vi "Xctrl interface-Set X axis multiplier.vi"(8 "error in (no error)":errorcluster) -> (0 "error out":errorcluster)   [LabVIEW 2020]
uses:
  XGrapher.xctl
  Global variables/gl_Functional Imaging-Global variables.vi
  SubVIs/Experiment header interface/Typedefs/Header file interface module functions enum.ctl
  Typedefs/Get-Set-Clear Control.ctl
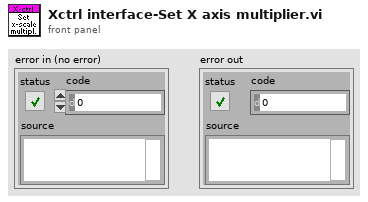
[diagram p1: front panel]
types:
  T1 = typedef "Get-Set-Clear Control.ctl" = enum16{"Get", "Set", "Clear"}
  T2 = typedef "Header file interface module functions enum.ctl" = enum16{"Load experiment header file", "Save experiment header file", "Clear stored values", "Read stored values", "Update specific value in memory", "Update values in memory"}
  T3 = typedef "Header parameters cluster-ALL.ctl" = cluster{"LOGIN":T4, "GLOBAL PARAMETERS":T5, "IMAGING MODES":T7, "TIME SERIES":T8, "MOTOR Z-STACK ":T11, "AOL Z-STACK":T12, "FUNCTIONAL IMAGING":T13, "VOLUME IMAGING":T13, "MOVEMENT CORRECTION":T17, "CALIBRATION":T19, "STATISTICS":T20, "BIOLOGY INFORMATION":T21, "Calibration Data":T22}
  T4 = typedef "Header params -Login.ctl" = cluster{"User":string, "Profile":string, "Software Version":string, "Experiment Date Time":timestamp}
  T5 = typedef "Header params-Global Parameters.ctl" = cluster{"MicroscopeID":string, "Microscope Type":string, "Objective":string, "Field of View (um)":dbl, "Fill time (us)":dbl, "Experiment Type":T6, "Stimuli Trigger":bool, "Speed Logging":bool}
  T6 = typedef "Experiment Type.ctl" = enum16{"In vivo", "In vitro", "Testing", "Calibration", "Other"}
  T7 = typedef "Header params-Imaging Modes.ctl" = cluster{"Time Series":bool, "Motor Zstack":bool, "AOL Zstack":bool, "Functional Imaging":bool, "Volume Imaging":bool}
  T8 = typedef "Header params-Time Series.ctl" = cluster{"Basic Image meta data":T9, "AOL z":dbl}
  T9 = typedef "Header params-Basic image meta data.ctl" = cluster{"Wavelength (nm)":dbl, "# averaged frames":dbl, "laser power (%)":dbl, "Pockels":dbl, "pixel dwell time (us)":dbl, "pmt 1":dbl, "pmt 2":dbl, "back apperture":dbl, "zoom":dbl, "field of view":dbl, "Frame Size":T10, "AOL x centre":dbl, "AOL y centre":dbl, "Stage x position":dbl, "Stage y position":dbl, "Stage z position":dbl}
  T10 = typedef "Frame Size.ctl" = u16
  T11 = typedef "Header params-Motor Z-stack.ctl" = cluster{"Hdr Basic Image meta data":T9, "Z Start":dbl, "Z Stop":dbl, "No of Planes":i32, "Laser Power (%) at Z Start":dbl, "Laser Power (%) at Z Stop":dbl}
  T12 = typedef "Header params-AOL Z-stack.ctl" = cluster{"Hdr Basic Image meta data":T9, "Z Start":dbl, "Z Stop":dbl, "No of Planes":i32, "Laser Power (%) at Z Start":dbl, "Laser Power (%) at Z Stop":dbl}
  T13 = typedef "Header params-Functional Imaging.ctl" = cluster{"Functional Mode":T14, "Variable Length":bool, "Variable Resolution":bool, "Pockels Modulation":bool, "Stimuli Trigger":bool, "Cool down enabled":bool, "AOL Mode":T15, "Plane Mode":T16, "Miniscan Dwell time per pixel (us)":dbl, "poi dwell time":dbl, "Number of trials":dbl, "Number of cycles":dbl, "Number of pois":dbl, "Number of miniscans":dbl, "Number of pixels in miniscan":dbl, "Rectangle ROI length":dbl, "Rectangle ROI height":dbl, "Frame rate (fps)":dbl, "Acquisition Length":dbl, "video length (sec)":dbl, "Stimuli delay (sec)":dbl, "Cool down time (sec)":dbl, "Basic Image meta data":T9, "Z Start (um)":dbl, "Z Stop (um)":dbl}
  T14 = typedef "Functional Mode.ctl" = enum16{"Point", "Line", "Patch", "Plane", "Volume"}
  T15 = typedef "AOL modes.ctl" = enum16{"Raster", "Structural", "Pointing", "Mini Scan", "Alignment"}
  T16 = typedef "Plane Mode.ctl" = u16
  T17 = typedef "Header params-Movement correction.ctl" = cluster{"Movement Correction":bool, "Axial Reference":bool, "Reference Source":T18, "Full Frame Size":dbl, "Reference Field of View":dbl, "Reference Zoom":dbl, "Reference dwell time (us)":dbl, "Reference X Pixels":dbl, "Reference Y Pixels":dbl, "Number of Z lines":dbl, "Size of Z pixels":dbl, "Axial Pixels":dbl, "Ignore Z lines":dbl, "Reference Scan Cycles":dbl, "Reference Threshold XY":dbl, "Reference Threshold Z":dbl, "Reference Average XY":dbl, "Reference Average Z":dbl, "Proportional Scale":dbl, "Integral Scale":dbl, "Proportional Scale Z":dbl, "Integral Scale Z":dbl, "Diff Threshold":dbl, "Diff Threshold Z":dbl, "Sliding Average":bool, "Reference count reset enabled":bool, "Scan Interval (ms)":dbl, "Ref Plot Refresh Rate (ms)":dbl}
  T18 = typedef "Reference source.ctl" = enum16{"Green channel", "Red channel"}
  T19 = typedef "Header params-Calibration Setup.ctl" = cluster{"Pockels Calibration File":path, "Calibration_ini file":path, "Setup_ini file":path}
  T20 = typedef "Header params-statistics.ctl" = cluster{"Z-stack duration (sec)":dbl, "Number of acquired data-points":dbl, "Acquisition time (ms)":dbl, "Number of acquired frames":dbl, "Intertrial times":dbl[]}
  T21 = typedef "Biology Information.ctl" = cluster{"Animal Code or Name":string, "Animal DoB":string, "Animal Age":string, "Animal Sex":string, "Animal Weight":string, "Date of Injection":string, "Date of Implant":string, "Site of Injection":string, "Animal Ear Notch":string, "AAV constructs":string, "Genetic background":string, "Optical reporter":string, "Region of brain imaged":string, "Other \ncomments":string}
  T22 = typedef "Header params-calibration data.ctl" = cluster{"Objective Name":string, "Calibration Wavelength":dbl, "Sum X":dbl, "Sum Y":dbl, "Diff X":dbl, "Diff Y":dbl, "Distortion Correction":dbl, " Z norm to um Scaling":dbl, " X norm to um Scaling":dbl}
  T23 = typedef "Functional Imging UI Refs.ctl" = cluster{"Menu ref":refnum<k9>, "Image control":refnum<vi>, "VI ref":refnum<vi>, "XGrapher":refnum<vi>, "Smoothing":refnum<vi>, "POI Averaging":refnum<vi>, "Normalize":refnum<vi>, "POI data points in each trial":refnum<vi>, "Channel":refnum<vi>, "Experiment data folder path":refnum<vi>, "[ROI vis]":refnum<vi>, "[Groups] visbl":T24, "Group Name":refnum<vi>, "POI index":refnum<vi>, "Trial No.":refnum<vi>, "Intensity Zoom":refnum<vi>, "Trial Cursor Enabled":refnum<vi>, "Number of Trials (ind 1)":refnum<vi>, "Number of Trials (ind 2)":refnum<vi>, "MiniScans Available":refnum<vi>, "POI Available":refnum<vi>, "Defer graph updates":refnum<vi>, "Waveform selector":refnum<vi>, "#of selected POI":refnum<vi>, "#of selected MiniScans":refnum<vi>, "#of selected groups":refnum<vi>, "Max Z-Projection":refnum<vi>, "Z-Plane Selector":refnum<vi>, "Index of miniscan point to visualise":refnum<vi>, "ROI vis. mode":refnum<vi>, "Total # of points":refnum<vi>, "Index of group clicked on":refnum<vi>, "Pane 1":refnum<vi>, "Pane 2":refnum<vi>, "Pane 3":refnum<vi>, "Pane 4":refnum<vi>, "Pane 5":refnum<vi>, "Pane 6":refnum<vi>, "Deselect all ROI":refnum<vi>, "Deselect all groups":refnum<vi>}
  T24 = typedef "Groups array referecne.ctl" = refnum<vi>
  T25 = typedef "XGrapher.xctl/Xctrl-Waveform graph ref.ctl" = refnum<vi>
  T26 = typedef "XGrapher.xctl/Xctrl-Timeline graph ref.ctl" = refnum<vi>
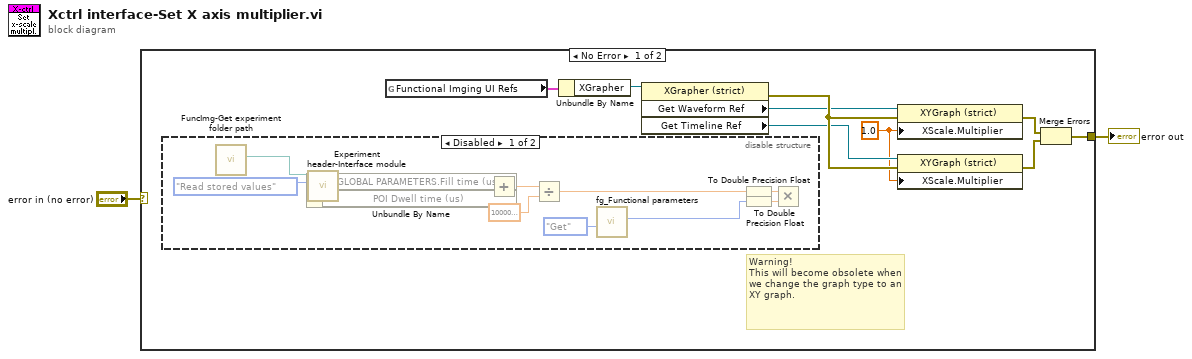
[diagram p0: block diagram]
diagram:
  n1 = case shown="No Error" "error in (no error)" {
    selector: "error in (no error)" -> [_ w24]
    tunnel: [w11 w24] -> w2
    frame No Error {
      w4 = 1.0 ("X Scale.Offset and Multiplier:Multiplier")
      # "Warning!\nThis will become obsolete when we change the graph type to an XY graph."
      n2 = disable-structure shown="Disabled" {
        frame Disabled {
          n3 = call "FuncImg-Get experiment folder path.vi"() -> ("Experiment data folder path"=w12:path)  [unwired: 10 in, 1 out]
          n4 = call "Experiment header-Interface module.vi"("Function"=Header_file_interface_module_functions_enum."Read stored values", "Experiment data folder path"=w12) -> ("All header parameters out"=w20:T3)  [unwired: 8 in, 1 out]
          n5 = Unbundle By Name(w20) -> ("GLOBAL PARAMETERS.Fill time (us)"=w14:dbl, "POI Dwell time (us)"=w15:dbl)
          n6 = Add(x=w14, y=w15) -> (x+y=w16:dbl)
          n7 = Divide(x=w16, y=sgl 1000000.0) -> (x/y=w18:dbl)
          n8 = call "fg_Functional parameters.vi"("Function"=Get-Set-Clear_Control."Get") -> ("# of ROI"=w23:i32)  [unwired: 7 in, 3 out]
          n9 = To Double Precision Float(number=w18) -> (double precision float=w19:dbl)
          n10 = To Double Precision Float(number=w23) -> (double precision float=w13:dbl)
          n11 = Multiply(x=w19, y=w13) -> ()  [unwired: 1 out]
        }
        frame Enabled {
        }
      }
      n12 = global read "gl_Functional Imaging-Global variables.vi" "Functional Imging UI Refs"() -> (w3:T23)
      n13 = Unbundle By Name(w3) -> ("XGrapher"=w8:refnum<vi>)
      n14 = property on="Property Node" class="XGrapher (strict)"(reference=w8) -> (error out=w7:errorcluster, "Get Waveform Ref"=w5:T25, "Get Timeline Ref"=w6:T26)  [unwired: 1 in, 1 out]
      n15 = property on="Property Node" class="XYGraph (strict)"(reference=w5, error in=w7, "XScale.Multiplier"=w4) -> (error out=w9:errorcluster)  [unwired: 1 out]
      n16 = property on="Property Node" class="XYGraph (strict)"(reference=w6, error in=w7, "XScale.Multiplier"=w4) -> (error out=w10:errorcluster)  [unwired: 1 out]
      n17 = Merge Errors(w9, w10) -> (w11:errorcluster)
    }
    frame Error {
    }
  }
  "error out" <- w2
